vi "waypoint_simple.vi"(6 "semaphore":T1, 7 "Motor Adress":T2(ring)=enum."3", 8 "error in (no error)":errorcluster, 9 "steps":i32, 10 "Direction (d)":i32(ring) items=["left", "right"], 11 "VISA ressource in":refnum<visa-resource-name>="COM1") -> (0 "error out":errorcluster={"status"=FALSE, "code"=1073676294, "source"="VISA Read in write_read.vi"}, 1 "Delta Steps":i32, 2 "Log File":string, 3 "VISA ressource out":refnum<visa-resource-name>)   [LabVIEW 2013]
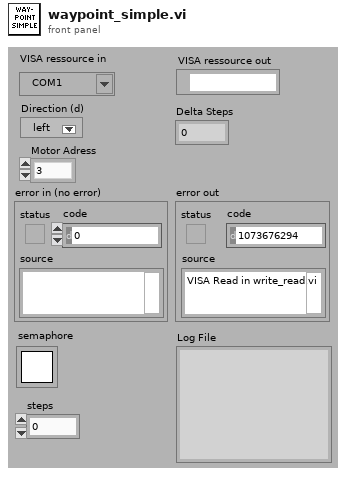
[diagram p1: front panel]
types:
  T1 = typedef "Semaphore RefNum" = refnum<k1>
  T2 = enum16{"All", "1", "2", "3", "4", "5", "6", "7", "8"}
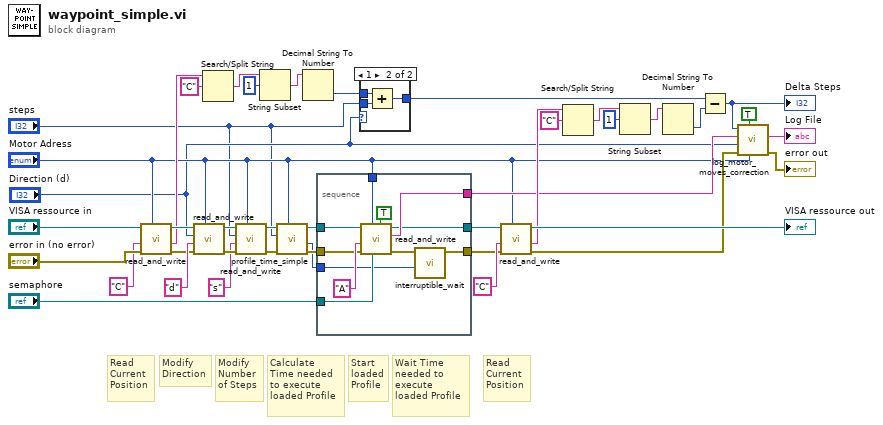
[diagram p0: block diagram]
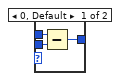
[diagram p2: hidden frame]
diagram:
  # "Modify\nNumber\nof Steps"
  # "Wait Time\nneeded to\nexecute\nloaded Profile"
  # "Read\nCurrent\nPosition"
  # "Start\nloaded\nProfile"
  # "Calculate\nTime needed\nto execute\nloaded Profile"
  # "Modify\nDirection"
  # "Read\nCurrent\nPosition"
  n1 = call "read_and_write.vi"("Motor Adress"="Motor Adress", "error in (no error)"="error in (no error)", "Command"="C", "VISA ressource in"="VISA ressource in") -> ("error out"=w38:errorcluster, "Answer"=w30:string, "VISA ressource out"=w37:refnum<visa-resource-name>)  [unwired: 4 in, 1 out]
  n2 = call "read_and_write.vi"("Motor Adress"="Motor Adress", "error in (no error)"=w38, "Command"="d", "value"="Direction (d)", "VISA ressource in"=w37) -> ("error out"=w11:errorcluster, "VISA ressource out"=w9:refnum<visa-resource-name>)  [unwired: 3 in, 2 out]
  n3 = Search/Split String(string=w30, search string/char (-)="C") -> (match + rest of string=w28:string)  [unwired: 1 in, 2 out]
  n4 = call "read_and_write.vi"("Motor Adress"="Motor Adress", "error in (no error)"=w11, "Command"="s", "value"="steps", "VISA ressource in"=w9) -> ("error out"=w10:errorcluster, "VISA ressource out"=w8:refnum<visa-resource-name>)  [unwired: 3 in, 2 out]
  n5 = String Subset(string=w28, offset (0)=1) -> (substring=w26:string)  [unwired: 1 in]
  n6 = call "profile_time_simple.vi"("Motor Adress"="Motor Adress", "error in (no error)"=w10, "steps in"="steps", "VISA ressource in"=w8) -> ("error out"=w33:errorcluster, "profile time (in ms)"=w17:u32, "VISA ressource out"=w34:refnum<visa-resource-name>)  [unwired: 3 in, 2 out]
  n7 = Decimal String To Number(string=w26) -> (number=w19:i32)  [unwired: 2 in, 1 out]
  n8 = stacked-sequence {
    tunnel: w34 -> [w51]
    tunnel: w33 -> [w50]
    tunnel: [w49] -> w14
    tunnel: "semaphore" -> [w48]
    tunnel: "Motor Adress" -> [w47]
    tunnel: [w43] -> w5
    tunnel: [w42] -> w4
    tunnel: w17 -> [w45]
    frame #0 {
      n9 = call "read_and_write.vi"("waypoint version"=TRUE, "semaphore"=w48, "Motor Adress"=w47, "error in (no error)"=w50, "Command"="A", "VISA ressource in"=w51) -> ("error out"=w44:errorcluster, "Log File (global)"=w49:string, "VISA ressource out"=w43:refnum<visa-resource-name>)  [unwired: 2 in, 1 out]
      n10 = call "interruptible_wait.vi"("profile_time"=w45, "Fehler (Eingang)"=w44) -> ("Fehler (Ausgang)"=w42:errorcluster)  [unwired: 9 in]
    }
  }
  n11 = case shown="1" "Direction (d)" {
    tunnel: w19 -> [w55 w58]
    tunnel: "steps" -> [w54 w57]
    tunnel: [w53 w56] -> w18
    frame 0, Default {
      n12 = Subtract(x=w55, y=w54) -> (x-y=w53:i32)
    }
    frame 1 {
      n13 = Add(x=w58, y=w57) -> (x+y=w56:i32)
    }
  }
  n14 = call "read_and_write.vi"("Motor Adress"="Motor Adress", "error in (no error)"=w4, "Command"="C", "VISA ressource in"=w5) -> ("error out"=w13:errorcluster, "Answer"=w21:string, "VISA ressource out"=→"VISA ressource out":refnum<visa-resource-name>)  [unwired: 4 in, 1 out]
  n15 = Search/Split String(string=w21, search string/char (-)="C") -> (match + rest of string=w23:string)  [unwired: 1 in, 2 out]
  n16 = String Subset(string=w23, offset (0)=1) -> (substring=w25:string)  [unwired: 1 in]
  n17 = Decimal String To Number(string=w25) -> (number=w20:i32)  [unwired: 2 in, 1 out]
  n18 = Subtract(x=w18, y=w20) -> (x-y=w16:i32)
  "Delta Steps" <- w16
  n19 = call "log_motor_moves_correction.vi"("Motor Adress"="Motor Adress", "waypoint version"=TRUE, "error in"=w13, "Direction"="Direction (d)", "Log File IN"=w14, "Delta Steps"=w16) -> ("error out"=→"error out":errorcluster, "Log File OUT"=→"Log File":string)  [unwired: 4 in]
